vi "To More Specific Class.vi"() -> ()   [LabVIEW 2023]
doc: "Illustrates how to use the To More Specific Class function to gain access to properties and methods specific to a particular class of object."
uses:
  <vilib>/Utility/traverseref.llb/TRef TravTarget.ctl
  <vilib>/Utility/traverseref.llb/VI Scripting - Traverse.lvlib
panel:
  out "Number of Tree Rows":i32[](array[numeric])
  out "Number of Multicolumn Listbox Rows":i32[](array[numeric])
  out "Number of Listbox Rows":i32[](array[numeric])
  out "All Control Labels in Target VI":string[](array[string])
  # "Overview: Demonstrates the use of the To More Specific Class function to read properties that are specific to a particular class of control.\nInstructions:\nRun the VI. It will count the number of rows in different control types on the front panel of a target VI."
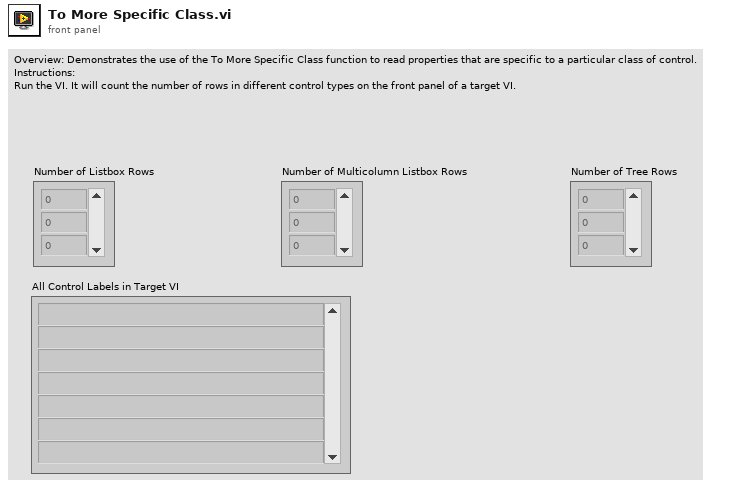
[diagram p1: front panel]
types:
  T1 = typedef "TRef TravTarget.ctl" = enum16{"FP", "BD", "Other"}
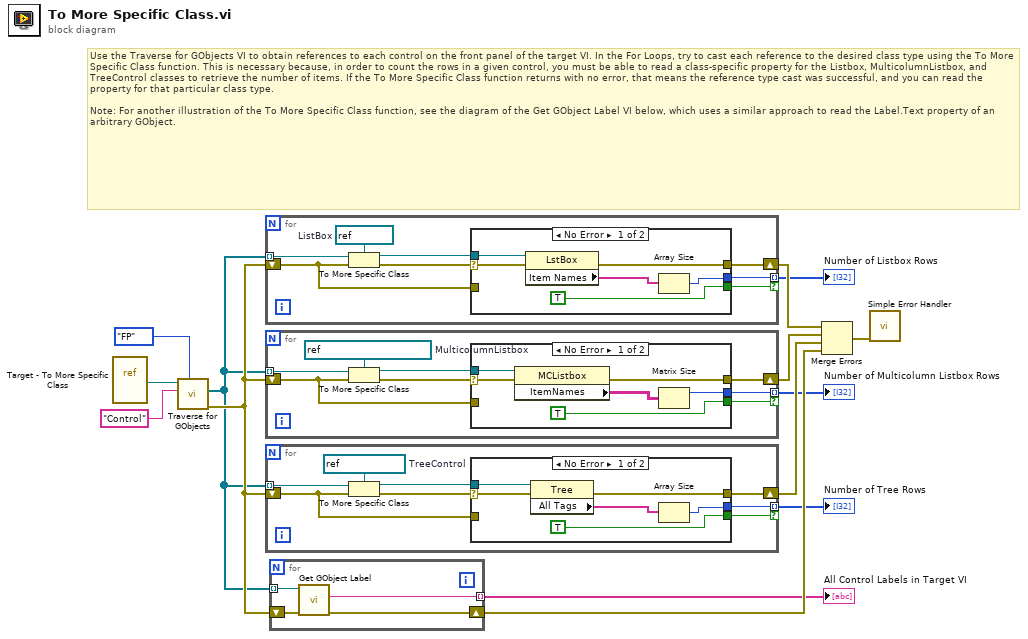
[diagram p0: block diagram]
diagram:
  # "Use the Traverse for GObjects VI to obtain references to each control on the front panel of the target VI. In the For Loops, try to cast each reference to the desired class type using the To More Specific Class function. This is necessary because, in order to count the rows in a given control, you must be able to read a class-specific property for the Listbox, MulticolumnListbox, and TreeControl classes to retrieve the number of items. If the To More Specific Class function returns with no error, that means the reference type cast was successful, and you can read the property for that particular class type.\n\nNote: For another illustration of the To More Specific Class function, see the diagram of the Get GObject Label VI below, which uses a similar approach to read the Label.Text property of an arbitrary GObject."
  n1 = vi-ref "Target - To More Specific Class.vi"() -> (w14:refnum<vi>)
  n2 = call <vilib>:"Traverse for GObjects.vi"("Traverse Target"=TRef_TravTarget."FP", "Class Name"="Control", "VI Refnum"=w14) -> ("error out"=w7:errorcluster, "References"=w6:refnum<vi>[])  [unwired: 5 in, 2 out]
  n3 = for {
    tunnel: w6 -> [w22] mode=indexing
    shift-right: [w18] -> w11
    shift-left: w7 -> [w15]
    tunnel: [w17] -> w1 mode=indexing if=w16
    w21 = refnum<vi> refnum  # ListBox
    n4 = To More Specific Class(target class=w21, reference=w22, error in=w15) -> (specific class reference=w19:refnum<vi>, error out=w20:errorcluster)
    n5 = case shown="No Error" w20 {
      selector: w20 -> [w28 _]
      tunnel: w19 -> [w27 _]
      tunnel: [w26 w29] -> w18
      tunnel: [w24 _] -> w17
      tunnel: [TRUE _] -> w16
      tunnel: w15 -> [_ w29]
      frame No Error {
        n6 = property class="LstBox"(reference=w27, error in=w28) -> (error out=w26:errorcluster, "Item Names"=w23:string[])  [unwired: 1 out]
        n7 = Array Size(array=w23) -> (size(s)=w24:i32)
      }
      frame Error {
      }
    }
  }
  "Number of Listbox Rows" <- w1
  n8 = for {
    tunnel: w6 -> [w37] mode=indexing
    shift-right: [w33] -> w10
    shift-left: w7 -> [w30]
    tunnel: [w32] -> w2 mode=indexing if=w31
    w36 = refnum<vi> refnum  # MulticolumnListbox
    n9 = To More Specific Class(target class=w36, reference=w37, error in=w30) -> (specific class reference=w34:refnum<vi>, error out=w35:errorcluster)
    n10 = case shown="No Error" w35 {
      selector: w35 -> [w43 _]
      tunnel: w34 -> [w42 _]
      tunnel: [w41 w44] -> w33
      tunnel: [w39 _] -> w32
      tunnel: [TRUE _] -> w31
      tunnel: w30 -> [_ w44]
      frame No Error {
        n11 = property class="MCListbox"(reference=w42, error in=w43) -> (error out=w41:errorcluster, "ItemNames"=w38:string[][])  [unwired: 1 out]
        n12 = Matrix Size(0:w38) -> (1:w39:i32)  [unwired: 1 out]
      }
      frame Error {
      }
    }
  }
  "Number of Multicolumn Listbox Rows" <- w2
  n13 = for {
    tunnel: w6 -> [w52] mode=indexing
    shift-right: [w48] -> w9
    shift-left: w7 -> [w45]
    tunnel: [w47] -> w3 mode=indexing if=w46
    w51 = refnum<vi> refnum  # TreeControl
    n14 = To More Specific Class(target class=w51, reference=w52, error in=w45) -> (specific class reference=w49:refnum<vi>, error out=w50:errorcluster)
    n15 = case shown="No Error" w50 {
      selector: w50 -> [w58 _]
      tunnel: w49 -> [w57 _]
      tunnel: [w56 w59] -> w48
      tunnel: [w54 _] -> w47
      tunnel: [TRUE _] -> w46
      tunnel: w45 -> [_ w59]
      frame No Error {
        n16 = property class="Tree"(reference=w57, error in=w58) -> (error out=w56:errorcluster, "All Tags"=w53:string[])  [unwired: 1 out]
        n17 = Array Size(array=w53) -> (size(s)=w54:i32)
      }
      frame Error {
      }
    }
  }
  "Number of Tree Rows" <- w3
  n18 = for {
    shift-right: [w61] -> w5
    shift-left: w7 -> [w63]
    tunnel: w6 -> [w62] mode=indexing
    tunnel: [w60] -> w4 mode=indexing
    n19 = call <vilib>:"Get GObject Label.vi"("error in (no error)"=w63, "GObject"=w62) -> ("error out"=w61:errorcluster, "Object Label"=w60:string)  [unwired: 5 in, 3 out]
  }
  "All Control Labels in Target VI" <- w4
  n20 = Merge Errors(w11, w10, w9, w5) -> (w8:errorcluster)
  n21 = call <vilib>:"Simple Error Handler.vi"("error in (no error)"=w8) -> ()  [unwired: 4 in, 5 out]
